vi "Write ActorRefContainer.vi"(8 "error in (no error)":errorcluster, 10 "ActorRefContainer":refnum<class "ActorRefContainer.lvclass">, 11 "ModuleAbstract in":refnum<class "ModuleAbstract.lvclass">) -> (0 "error out":errorcluster, 3 "ModuleAbstract out":refnum<class "ModuleAbstract.lvclass">)   [LabVIEW 2019, in "ModuleAbstract.lvlib" / "ModuleAbstract.lvclass"]
uses:
  ModuleAbstract.lvclass
  Containers/ActorRefContainer/ActorRefContainer.lvclass
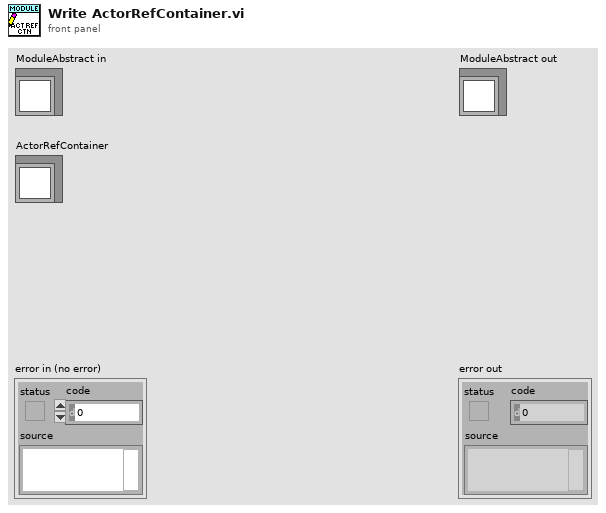
[diagram p1: front panel]
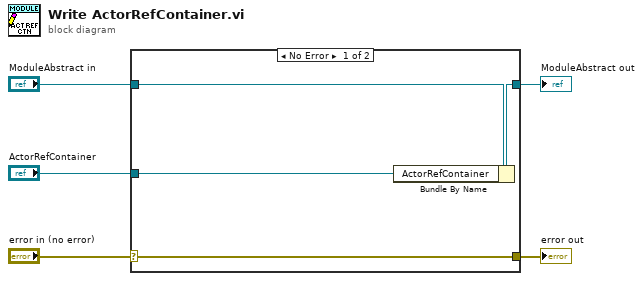
[diagram p0: block diagram]
diagram:
  n1 = case shown="No Error" "error in (no error)" {
    selector: "error in (no error)" -> [w9 w10]
    tunnel: [w9 w10] -> w4
    tunnel: [w7 w11] -> w2
    tunnel: "ModuleAbstract in" -> [w8 w11]
    tunnel: "ActorRefContainer" -> [w6 _]
    frame No Error {
      n2 = Bundle By Name(cluster=w8, "ActorRefContainer"=w6) -> (w7:refnum<class "ModuleAbstract.lvclass">)
    }
    frame Error {
    }
  }
  "error out" <- w4
  "ModuleAbstract out" <- w2
